vi "MDAQ_ReadoldCSVfile.vi"(8 "error in":errorcluster, 11 "file path (use dialog)":path) -> (0 "error out":errorcluster, 1 "Run Data Cluster":T1 {"Temperature B" scale=0.0..100.0; "Temperature A" scale=0.0..100.0}, 2 "Run Info Out":T2)   [LabVIEW 2021]
uses:
  XML_Cluster.ctl
  DAT_Cluster.ctl
  <vilib>/Utility/error.llb/DialogType.ctl
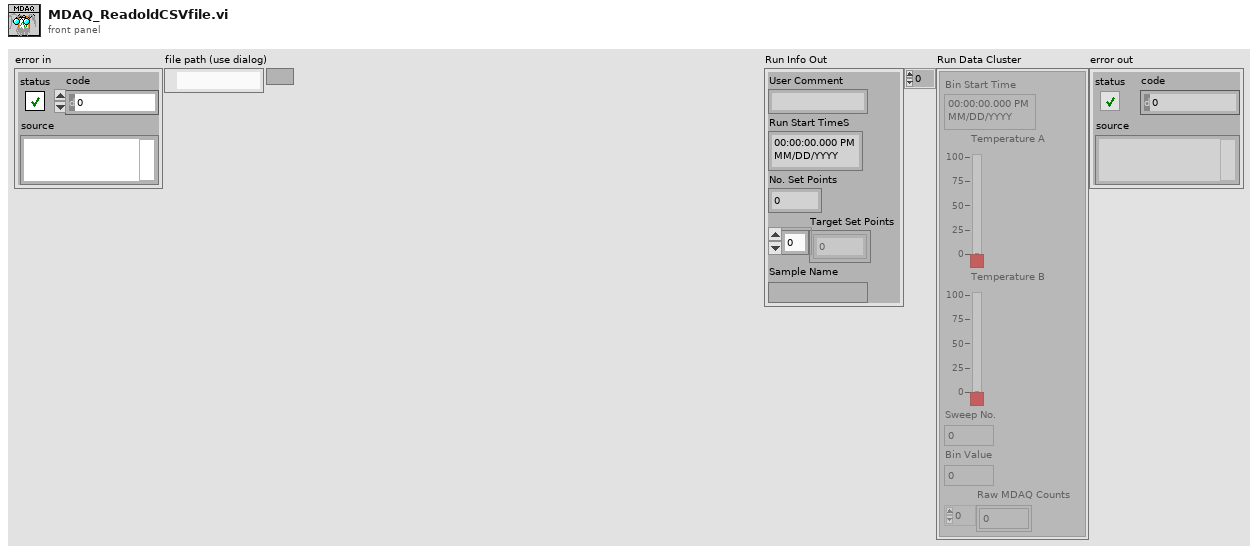
[diagram p1: front panel]
types:
  T1 = typedef "DAT_Cluster.ctl" = cluster{"Bin Start Time":timestamp, "Temperature A":dbl, "Temperature B":dbl, "Sweep No.":i32, "Bin Value":i32, "Raw MDAQ Counts":i32[]}[]
  T2 = typedef "XML_Cluster.ctl" = cluster{"User Comment":string, "Run Start TimeS":timestamp, "No. Set Points":u32, "Target Set Points":i32[], "Sample Name":string}
  T3 = typedef "DialogType.ctl" = u16
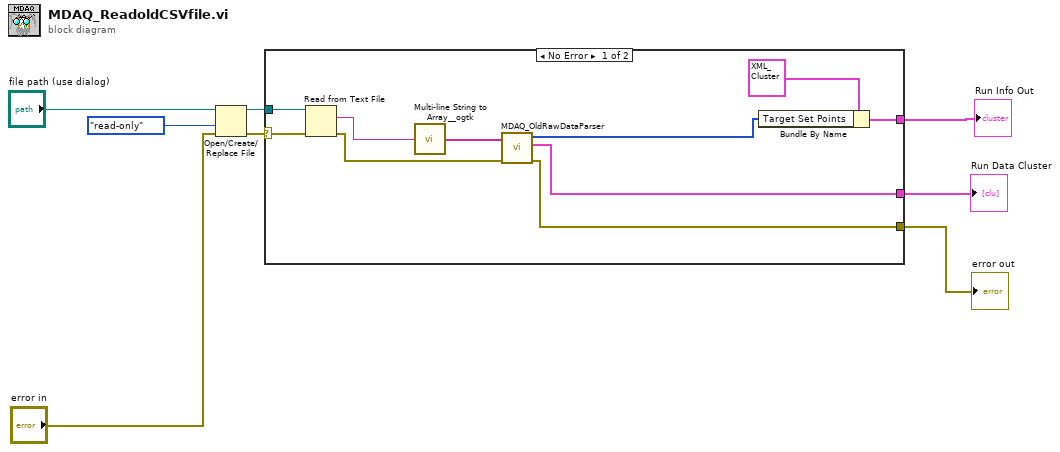
[diagram p0: block diagram]
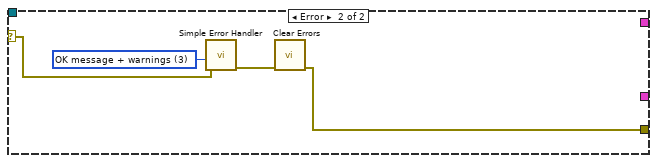
[diagram p2: hidden frame]
diagram:
  n1 = Open/Create/Replace File(file path (use dialog)="file path (use dialog)", error in="error in", access (0:read/write)=enum16{"read/write", "read-only", "write-only"}."read-only") -> (refnum out=w4:refnum<file>, error out=w5:errorcluster)  [unwired: 3 in, 1 out]
  n2 = case shown="No Error" w5 {
    selector: w5 -> [w17 w21]
    tunnel: w4 -> [w18 _]
    tunnel: [w14 _] -> w3
    tunnel: [w13 w19] -> w2
    tunnel: [w10 _] -> w1
    frame No Error {
      n3 = Read from Text File(file (use dialog)=w18, error in=w17) -> (text=w16:string, error out=w12:errorcluster)  [unwired: 2 in, 2 out]
      n4 = call <userlib>:"Multi-line String to Array__ogtk.vi"("string"=w16) -> ("lines"=w15:string[])
      n5 = call "MDAQ_OldRawDataParser.vi"("error in"=w12, "Raw Data In"=w15) -> ("error out"=w13:errorcluster, "Run Data Cluster"=w14:T1, "SetPoints array"=w9:i32[])  [unwired: 7 in]
      n6 = Bundle By Name(cluster=T2 {"User Comment"="", "Run Start TimeS"=timestamp(0 s since 1904-01-01), "No. Set Points"=0, "Target Set Points"=[], "Sample Name"=""} ("Run Info Out"), "Target Set Points"=w9) -> (w10:T2)
    }
    frame Error {
      w22 = T3 3 items=["no dialog", "OK message", "continue or stop message", "OK message + warnings", "continue/stop + warnings"] ("type of dialog (OK msg:1)")
      n7 = call <vilib>:"Simple Error Handler.vi"("type of dialog (OK msg:1)"=w22, "error in (no error)"=w21) -> ("error out"=w20:errorcluster)  [unwired: 3 in, 4 out]
      n8 = call <vilib>:"Clear Errors.vi"("error in (no error)"=w20) -> ("error out"=w19:errorcluster)  [unwired: 5 in, 1 out]
    }
  }
  "Run Data Cluster" <- w3
  "Run Info Out" <- w1
  "error out" <- w2
